vi "OmronFinsNET.vi"() -> ()   [LabVIEW 2016]
uses:
  C:/Users/Administrator/Desktop/HslCommunicationDemo-v5.7.0/HslCommunication.dll
  HslCommunication.dll
panel:
  in  "读写地址":string="D414"
  out "读取成功":bool
  out "连接成功":bool
  in  "读写次数":i32=100
  out "单次读写时间":u32 format="%.0fms"
  out "写入成功":bool
  out "总时间":u32 format="%.0fms"
  out "读写值":i16
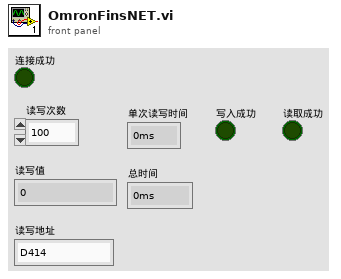
[diagram p1: front panel]
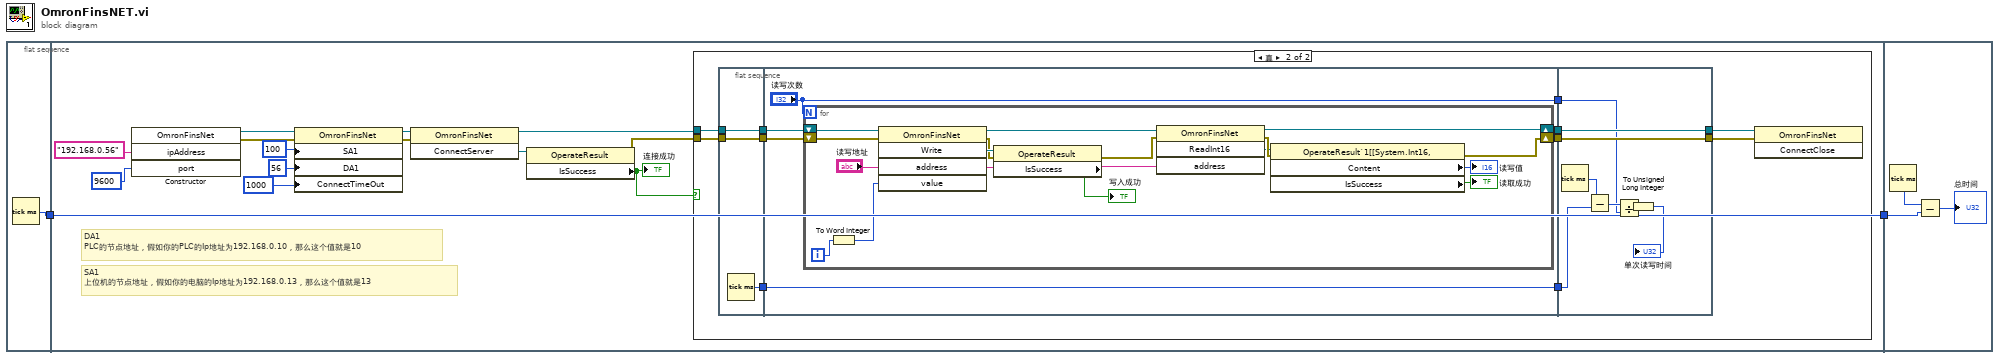
[diagram p0: block diagram]
diagram:
  n1 = flat-sequence {
    tunnel: [w3] -> w2
    tunnel: w2 -> [w15]
    tunnel: [w15] -> w1
    tunnel: w1 -> [w62]
    frame #0 {
      n2 = Tick Count (ms)() -> (millisecond timer value=w3:u32)
    }
    frame #1 {
      # "SA1 \n上位机的节点地址，假如你的电脑的Ip地址为192.168.0.13，那么这个值就是13"
      # "DA1 \nPLC的节点地址，假如你的PLC的Ip地址为192.168.0.10，那么这个值就是10"
      n3 = constructor class="OmronFinsNet"("ipAddress"="192.168.0.56", "port"=9600) -> (reference out=w4:refnum<k24>, error out=w9:errorcluster)  [unwired: 3 in, 3 out]
      n4 = property class="OmronFinsNet"(reference=w4, error in=w9, "SA1"=u8 100, "DA1"=u8 56, "ConnectTimeOut"=1000) -> (reference out=w11:refnum<k24>, error out=w10:errorcluster)
      n5 = invoke class="OmronFinsNet" method="ConnectServer"(reference=w11, error in=w10) -> (reference out=w14:refnum<k24>, "ConnectServer"=w6:refnum<k24>)  [unwired: 1 in, 1 out]
      n6 = property class="OperateResult"(reference=w6) -> (error out=w13:errorcluster, "IsSuccess"=w12:bool)  [unwired: 1 in, 1 out]
      "连接成功" <- w12
      n7 = case shown="真" w12 {
        tunnel: w14 -> [_ w21]
        tunnel: w13 -> [_ w20]
        frame False {
        }
        frame True {
          n8 = flat-sequence {
            tunnel: w20 -> [w30]
            tunnel: w21 -> [w31]
            tunnel: [w31] -> w28
            tunnel: [w30] -> w27
            tunnel: [w29] -> w26
            tunnel: w28 -> [w37]
            tunnel: w27 -> [w36]
            tunnel: [w35] -> w25
            tunnel: [w34] -> w24
            tunnel: [w33] -> w23
            tunnel: w26 -> [w33]
            tunnel: ["读写次数"] -> w22
            tunnel: [w60] -> w18
            tunnel: [w61] -> w19
            tunnel: w25 -> [w61]
            tunnel: w24 -> [w60]
            tunnel: w23 -> [w58]
            tunnel: w22 -> [w56]
            frame #0 {
              n9 = Tick Count (ms)() -> (millisecond timer value=w29:u32)
            }
            frame #1 {
              n10 = for {
                N: "读写次数" -> [_]
                shift-right: [w39] -> w35
                shift-left: w37 -> [w42]
                shift-right: [w38] -> w34
                shift-left: w36 -> [w52]
                i -> [w51]
                n11 = To Word Integer(number=w51) -> (16bit integer=w50:i16)
                n12 = invoke class="OmronFinsNet" method="Write"(reference=w42, error in=w52, "address"="读写地址", "value"=w50) -> (reference out=w41:refnum<k24>, error out=w43:errorcluster, "Write"=w49:refnum<k24>)  [unwired: 1 in, 2 out]
                n13 = property class="OperateResult"(reference=w49, error in=w43) -> (error out=w40:errorcluster, "IsSuccess"=→"写入成功":bool)  [unwired: 1 out]
                n14 = invoke class="OmronFinsNet" method="ReadInt16"(reference=w41, error in=w40, "address"="读写地址") -> (reference out=w39:refnum<k24>, error out=w47:errorcluster, "ReadInt16"=w46:refnum<k24>)  [unwired: 1 in, 1 out]
                n15 = property class="OperateResult`1[[System.Int16, "(reference=w46, error in=w47) -> (error out=w38:errorcluster, "Content"=→"读写值":i16, "IsSuccess"=→"读取成功":bool)  [unwired: 1 out]
              }
            }
            frame #2 {
              n16 = Tick Count (ms)() -> (millisecond timer value=w59:u32)
              n17 = Subtract(x=w59, y=w58) -> (x-y=w57:u32)
              n18 = Divide(x=w57, y=w56) -> (x/y=w55:dbl)
              n19 = To Unsigned Long Integer(number=w55) -> (unsigned 32bit integer=→"单次读写时间":u32)
            }
          }
          n20 = invoke class="OmronFinsNet" method="ConnectClose"(reference=w19, error in=w18) -> ()  [unwired: 1 in, 3 out]
        }
      }
    }
    frame #2 {
      n21 = Tick Count (ms)() -> (millisecond timer value=w63:u32)
      n22 = Subtract(x=w63, y=w62) -> (x-y=→"总时间":u32)
    }
  }
